vi "Actor Core.vi"(8 "error in":errorcluster, 11 "IMAQ Display in":refnum<class "HIJ Vision Display.lvclass">) -> (0 "error out":errorcluster, 3 "Actor out":refnum<class "Actor.lvclass">)   [LabVIEW 2014, in "HIJ Vision Display.lvlib" / "HIJ Vision Display.lvclass"]
doc: "(<B>Filename</B>: Actor Framework.lvlib:Actor.lvclass:Actor Core.vi)\n\nReceives messages to the actor, reacts to them, and initiates any error handling that may shut the actor down.\n\nDescendant classes may override this VI to append parallel tasks for the actor to complete while it handles messages. Overrides use the Call Parent Method node."
uses:
  HIJ Vision Display.lvclass
  <vilib>/ActorFramework/Actor/Actor.lvclass
  Palette.ctl
  Shared Code/Viewable Actor/ViewableActor/ViewableActor.lvclass/ViewableActor.ctl
  HIJ Vision Display.lvclass/HIJ Vision Display.ctl
  <vilib>/ActorFramework/Actor/Actor.lvclass/Actor.ctl
  <vilib>/ActorFramework/Message Enqueuer/Message Enqueuer.lvclass/Message Enqueuer.ctl
  HIJ Vision Display Messages/Write ROI Msg/Write ROI Msg.lvclass/Write ROI Msg.ctl
  HIJ Vision Display Messages/Send Reply Actor State/Send Reply Actor State.lvclass
  <vilib>/ActorFramework/Reply Msg/Reply Msg.lvclass/Reply Msg.ctl
  HIJ Vision Display Messages/Contex Menu Selection Msg/Contex Menu Selection Msg.lvclass/Contex Menu Selection Msg.ctl
  Shared Code/Viewable Actor/ViewableActor/Write UI VI Ref.vi
  <vilib>/ActorFramework/Message Enqueuer/Init from Existing Queue.vi
  <vilib>/ActorFramework/Message Enqueuer/Enqueue.vi
  <vilib>/ActorFramework/Message Priority Queue/Priority Enqueue.vi
  <vilib>/ActorFramework/Message Enqueuer/Message Enqueuer.lvclass
  HIJ Vision Display Messages/Write ROI Msg/Write ROI Msg.lvclass
  HIJ Vision Display Messages/Evaluate with new Params Msg/Evaluate with new Params Msg.lvclass
  HIJ Vision Display Messages/Contex Menu Selection Msg/Contex Menu Selection Msg.lvclass
  Shared Code/Viewable Actor/ViewableActor/ViewableActor.lvclass
  Utility/POLARIS Vision utility.lvlib
  <vilib>/ActorFramework/Reply Msg/Reply Msg.lvclass
  HIJ Vision Display Messages/Show Select Report File Dialog Msg/Show Select Report File Dialog Msg.lvclass
  HIJ Vision Display Messages/Delete ROI Msg/Delete ROI Msg.lvclass
  HIJ Vision Display Messages/Show Display Settings Dialog Msg/Show Display Settings Dialog Msg.lvclass
  HIJ Vision Display Messages/New ROI and Overlay Selection Msg/New ROI and Overlay Selection Msg.lvclass
  HIJ Vision Display Messages/Show ROI Name Dialog Msg/Show ROI Name Dialog Msg.lvclass
  HIJ Vision Display Messages/Save Image Msg/Save Image Msg.lvclass
  HIJ Vision Display Messages/Show Report Msg/Show Report Msg.lvclass
  HIJ Vision Display Messages/Show Image Source Settings Msg/Show Image Source Settings Msg.lvclass
panel:
  in  "Zoom Buttons":enum32{"Zoom in", "Zoom out", "Center"}(radio)
  out "Image":T1(plugin-control)
  in  "StopSignal":bool=TRUE
  in  "Pallete":T2={"Teiler"=1, "Palette Type"=0} {"Teiler" min=1 max=5; "Palette Type" items=["Grayscale", "Binary", "Gradient", "Rainbow", "Temperature", "User Defined"]}
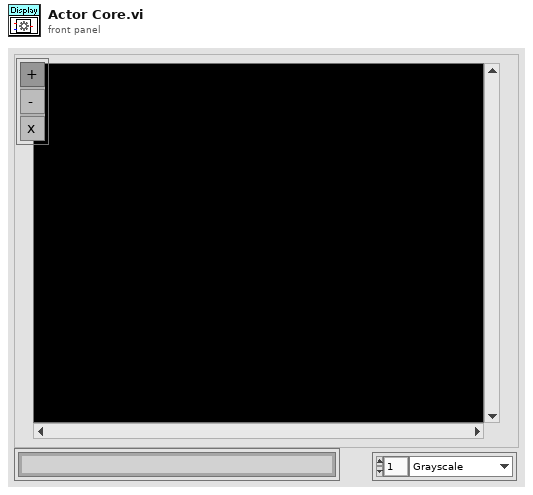
[diagram p1: front panel]
types:
  T1 = typedef "IMAQ Image.ctl" = refnum<image>
  T2 = typedef "HIJ Vision Display.lvlib/HIJ Vision Display.lvclass/Palette.ctl" = cluster{"Teiler":i32, "Palette Type":u32}
  T3 = typedef "ROI Descriptor" = cluster{"Global Rectangle":i32[], "Contours":cluster{"ID":enum32{"External", "Internal"}, "Type":u32, "Coordinates":i32[]}[]}
  T4 = cluster{"Global Rectangle":i32[], "Contours":cluster{"Contour Type":u32, "ROI Type":u32, "Points":i32[]}[]}
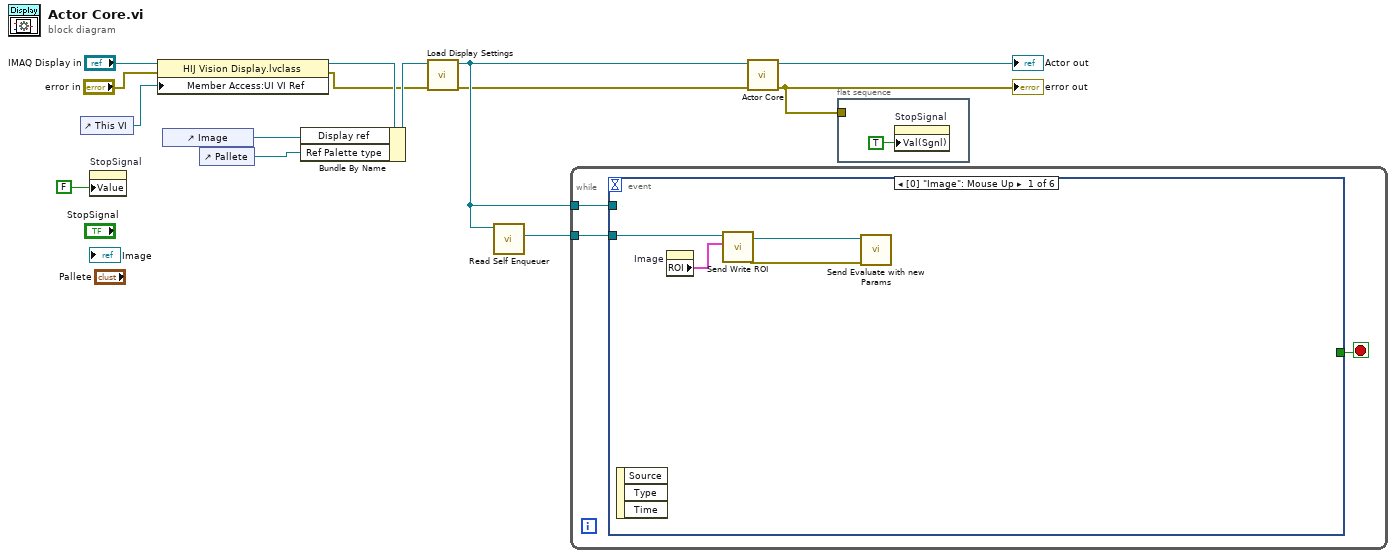
[diagram p0: block diagram]
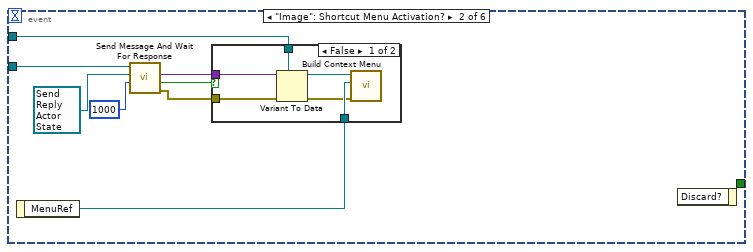
[diagram p2: hidden frame]
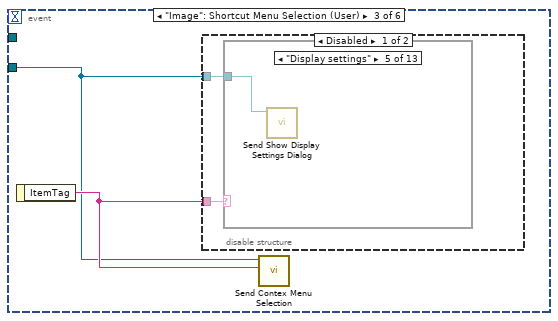
[diagram p4: hidden frame]
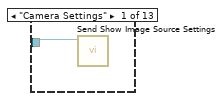
[diagram p5: hidden frame]
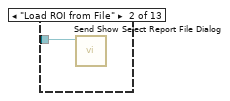
[diagram p6: hidden frame]
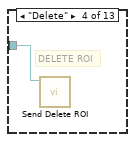
[diagram p8: hidden frame]
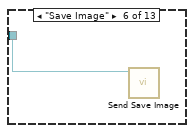
[diagram p9: hidden frame]
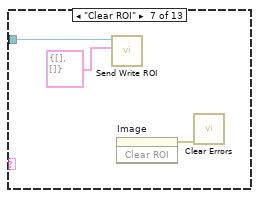
[diagram p10: hidden frame]
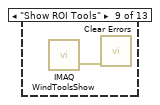
[diagram p12: hidden frame]
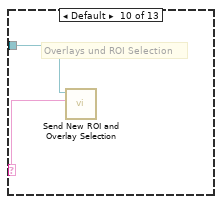
[diagram p13: hidden frame]
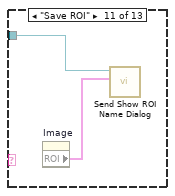
[diagram p14: hidden frame]
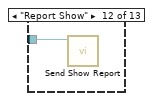
[diagram p15: hidden frame]
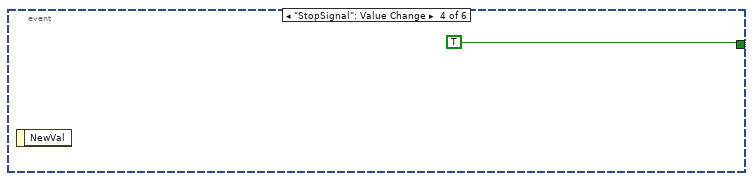
[diagram p18: hidden frame]
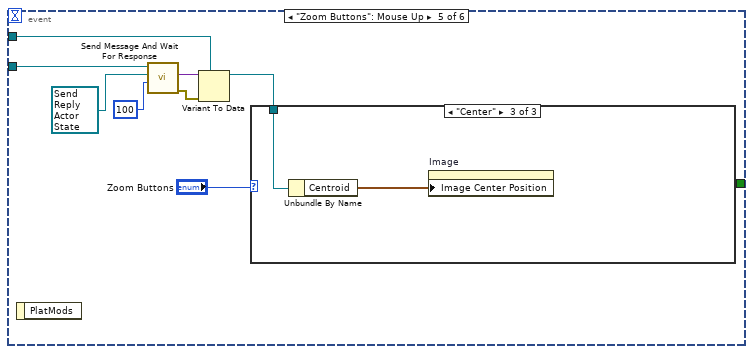
[diagram p19: hidden frame]
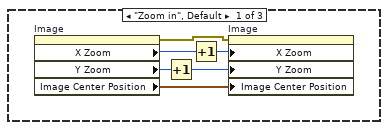
[diagram p20: hidden frame]
diagram:
  n1 = control-ref of="This VI"() -> (w7:refnum<vi>)
  n2 = property on="StopSignal" class="Bool (strict)"("Value"=FALSE ("Value (Signaling)")) -> ()  [unwired: 2 in, 2 out]
  n3 = property class="HIJ Vision Display.lvclass"(reference="IMAQ Display in", error in="error in", "Member Access:UI VI Ref"=w7) -> (reference out=w8:refnum<class "HIJ Vision Display.lvclass">, error out=w3:errorcluster)
  n4 = control-ref of="Image"() -> (w9:refnum<vi>)
  n5 = control-ref of="Pallete"() -> (w5:refnum<vi>)
  n6 = Bundle By Name(cluster=w8, "Display ref"=w9, "Ref Palette type"=w5) -> (w10:refnum<class "HIJ Vision Display.lvclass">)
  n7 = call-dynamic "Load Display Settings.vi"("error in (no error)"=w3, "AF IMAQ Display in"=w10) -> ("error out"=w2:errorcluster, "AF IMAQ Display out"=w4:refnum<class "HIJ Vision Display.lvclass">)  [unwired: 8 in]
  n8 = call <vilib>:"Read Self Enqueuer.vi"("Actor"=w4) -> ("Self Enqueuer"=w1:refnum<class "Message Enqueuer.lvclass">)  [unwired: 10 in]
  n9 = while {
    tunnel: w1 -> [w17]
    tunnel: w4 -> [w16]
    stop <- w15 stop-if-true
    n10 = event shown="[0] \"Image\": Mouse Up" {
      selector: _ -> [_ _ _ _ _ _]
      dyn-events: _ -> [_ _ _ _ _ _]
      timeout: _ -> [_ _ _ _ _ _]
      tunnel: w17 -> [w21 w27 w36 _ w56 _]
      tunnel: w16 -> [_ w29 _ _ w55 _]
      tunnel: [_ _ _ TRUE _ _] -> w15
      event "Image": Mouse Up {
        n11 = event-data() -> ()  [unwired: 1 in, 3 out]
        n12 = property on="Image" class="ImageControl"() -> ("ROI"=w20:T4)  [unwired: 2 in, 2 out]
        n13 = call "Send Write ROI.vi"("ROI Descriptor"=w20, "Message Enqueuer"=w21) -> ("error out"=w18:errorcluster, "Message Enqueuer out"=w19:refnum<class "Message Enqueuer.lvclass">)  [unwired: 8 in]
        n14 = call "Send Evaluate with new Params.vi"("error in (no error)"=w18, "Message Enqueuer"=w19) -> ()  [unwired: 8 in, 2 out]
      }
      event "Image": Shortcut Menu Activation? {
        n15 = event-data() -> ("MenuRef"=w28:refnum<k9>)  [unwired: 1 in]
        n16 = call <vilib>:"Send Message And Wait For Response.vi"("timeout in ms (-1)"=1000, "Original Message"=refnum<class "Send Reply Actor State.lvclass"> refnum ("IMAQ Display.lvlib:Send Reply Actor State.lvclass"), "Message Enqueuer in"=w27) -> ("error out"=w26:errorcluster, "timed out?"=w22:bool, "Reply"=w25:variant)  [unwired: 5 in, 1 out]
        n17 = case shown="False" w22 {
          tunnel: w26 -> [w35 _]
          tunnel: w25 -> [w34 _]
          tunnel: w29 -> [w33 _]
          tunnel: w28 -> [w32 _]
          frame False {
            n18 = Variant To Data(error in=w35, type=w33, Variant=w34) -> (data=w30:refnum<class "HIJ Vision Display.lvclass">, error out=w31:errorcluster)
            n19 = call-dynamic "Build Context Menu.vi"("error in (no error)"=w31, "MenuRef"=w32, "HIJ Vision Display in"=w30) -> ()  [unwired: 6 in, 3 out]
          }
          frame True {
          }
        }
        n20 = event-data() -> ()  [unwired: 2 in, 1 out]
      }
      event "Image": Shortcut Menu Selection (User) {
        n21 = event-data() -> ("ItemTag"=w37:string)  [unwired: 1 in]
        n22 = disable-structure shown="Disabled" {
          disable-tunnel: w37 -> [w39 _]
          disable-tunnel: w36 -> [w38 _]
          frame Disabled {
            n23 = case shown="\"Display settings\"" w39 {
              selector: w39 -> [_ _ _ _ _ _ _ _ _ w49 _ _ _]
              tunnel: w38 -> [w40 w41 _ w42 w43 w44 w46 _ _ w50 w52 w53 _]
              frame "Camera Settings" {
                n24 = call "Send Show Image Source Settings.vi"("Message Enqueuer"=w40) -> ()  [unwired: 9 in, 2 out]
              }
              frame "Load ROI from File" {
                n25 = call "Send Show Select Report File Dialog.vi"("Message Enqueuer"=w41) -> ()  [unwired: 9 in, 2 out]
              }
              frame "Save background" {
                # "#BGImage"
              }
              frame "Delete" {
                # "DELETE ROI"
                n26 = call "Send Delete ROI.vi"("Message Enqueuer"=w42) -> ()  [unwired: 9 in, 2 out]
              }
              frame "Display settings" {
                n27 = call "Send Show Display Settings Dialog.vi"("Message Enqueuer"=w43) -> ()  [unwired: 9 in, 2 out]
              }
              frame "Save Image" {
                n28 = call "Send Save Image.vi"("Message Enqueuer"=w44) -> ()  [unwired: 9 in, 2 out]
              }
              frame "Clear ROI" {
                n29 = call "Send Write ROI.vi"("ROI Descriptor"=T3 {"Global Rectangle"=[], "Contours"=[]}, "Message Enqueuer"=w46) -> ()  [unwired: 8 in, 2 out]
                n30 = invoke on="Image" class="ImageControl" method="Clear ROI"() -> (error out=w47:errorcluster)  [unwired: 3 in, 2 out]
                n31 = call <vilib>:"Clear Errors.vi"("error in (no error)"=w47) -> ()  [unwired: 5 in, 2 out]
              }
              frame "Substract BG" {
              }
              frame "Show ROI Tools" {
                n32 = call "IMAQ WindToolsShow"() -> ("error out"=w48:errorcluster)  [unwired: 5 in, 1 out]
                n33 = call <vilib>:"Clear Errors.vi"("error in (no error)"=w48) -> ()  [unwired: 5 in, 2 out]
              }
              frame Default {
                # "Overlays und ROI Selection"
                n34 = call "Send New ROI and Overlay Selection.vi"("ItemTag"=w49, "Message Enqueuer"=w50) -> ()  [unwired: 8 in, 2 out]
              }
              frame "Save ROI" {
                n35 = property on="Image" class="ImageControl"() -> ("ROI"=w51:T4)  [unwired: 2 in, 2 out]
                n36 = call "Send Show ROI Name Dialog.vi"("ROI Descriptor"=w51, "Message Enqueuer"=w52) -> ()  [unwired: 8 in, 2 out]
              }
              frame "Report Show" {
                n37 = call "Send Show Report.vi"("Message Enqueuer"=w53) -> ()  [unwired: 9 in, 2 out]
              }
              frame "Report Load" {
              }
            }
          }
          frame Enabled {
          }
        }
        n38 = call "Send Contex Menu Selection.vi"("MenuItem"=w37, "Message Enqueuer"=w36) -> ()  [unwired: 8 in, 2 out]
      }
      event "StopSignal": Value Change {
        n39 = event-data() -> ()  [unwired: 1 in, 1 out]
      }
      event "Zoom Buttons": Mouse Up {
        n40 = event-data() -> ()  [unwired: 1 in, 1 out]
        n41 = call <vilib>:"Send Message And Wait For Response.vi"("timeout in ms (-1)"=100, "Original Message"=refnum<class "Send Reply Actor State.lvclass"> refnum ("IMAQ Display.lvlib:Send Reply Actor State.lvclass"), "Message Enqueuer in"=w56) -> ("error out"=w61:errorcluster, "Reply"=w60:variant)  [unwired: 5 in, 2 out]
        n42 = Variant To Data(error in=w61, type=w55, Variant=w60) -> (data=w57:refnum<class "HIJ Vision Display.lvclass">)  [unwired: 1 out]
        n43 = case shown="\"Center\"" "Zoom Buttons" {
          tunnel: w57 -> [_ _ w85]
          frame "Zoom in", Default {
            n44 = property on="Image" class="ImageControl"() -> (error out=w63:errorcluster, "X Zoom"=w64:i32, "Y Zoom"=w65:i32, "Image Center Position"=w68:cluster{"X":u32, "Y":u32})  [unwired: 2 in, 1 out]
            n45 = Increment(x=w65) -> (x+1=w67:i32)
            n46 = Increment(x=w64) -> (x+1=w66:i32)
            n47 = property on="Image" class="ImageControl"(error in=w63, "X Zoom"=w66, "Y Zoom"=w67, "Image Center Position"=w68) -> ()  [unwired: 1 in, 2 out]
          }
          frame "Zoom out" {
            n48 = property on="Image" class="ImageControl"() -> (error out=w69:errorcluster, "X Zoom"=w74:i32, "Y Zoom"=w73:i32, "Image Center Position"=w70:cluster{"X":u32, "Y":u32})  [unwired: 2 in, 1 out]
            n49 = Decrement(x=w74) -> (x-1=w76:i32)
            n50 = Decrement(x=w73) -> (x-1=w75:i32)
            n51 = case shown="0" w76 {
              selector: w76 -> [w80 w83]
              tunnel: w75 -> [w81 w82]
              tunnel: [w79 w83] -> w72
              tunnel: [w78 w82] -> w71
              frame 0 {
                w77 = 2 ("x")
                n52 = Subtract(x=w80, y=w77) -> (x-y=w79:i32)
                n53 = Subtract(x=w81, y=w77) -> (x-y=w78:i32)
              }
              frame 1, Default {
              }
            }
            n54 = property on="Image" class="ImageControl"(error in=w69, "X Zoom"=w72, "Y Zoom"=w71, "Image Center Position"=w70) -> ()  [unwired: 1 in, 2 out]
          }
          frame "Center" {
            n55 = Unbundle By Name(w85) -> ("Centroid"=w84:cluster{"X Centroid":sgl, "Y Centroid":sgl})
            n56 = property on="Image" class="ImageControl"("Image Center Position"=w84) -> ()  [unwired: 2 in, 2 out]
          }
        }
      }
      event Value Change {
        n57 = event-data() -> ("NewVal.Palette Type"=w87:u32, "NewVal.Teiler"=w88:i32)  [unwired: 1 in]
        n58 = call "UserPalette-xRainbows.vi"("Teiler"=w88) -> ("Array"=w86:cluster{u8, u8, u8}[])  [unwired: 1 in]
        n59 = property on="Image" class="ImageControl"("Palette Type"=w87, "User Palette"=w86) -> ()  [unwired: 2 in, 2 out]
      }
    }
  }
  n60 = call-parent "Actor Core.vi"("error in"=w2, "Actor in"=w4) -> ("error out"=w12:errorcluster, "Actor out"=→"Actor out":refnum<class "Actor.lvclass">)  [unwired: 8 in]
  "error out" <- w12
  n61 = flat-sequence {
    tunnel: w12 -> [_]
    frame #0 {
      n62 = property on="StopSignal" class="Bool (strict)"("Val(Sgnl)"=TRUE ("Value (Signaling)")) -> ()  [unwired: 2 in, 2 out]
    }
  }
